vi "PH_Cam_BaseClass.ProcEvents.vi"(0 "i ref in":refnum<vi>, 5 "error in":errorcluster) -> (14 "i ref out":refnum<vi>, 19 "error out":errorcluster)   [LabVIEW 2014, in "PH_Cam_BaseClass.lvlib"]
doc: "This method is used to define the events the object will listen to. Add your own events here."
uses:
  PH_Cam_BaseClass.lvlib
  CS_Core/BaseProcess/BaseProcess.event definition.ctl
  CS_Core/CAEObj/CAEObj.event definition.ctl
  CS_Core/BaseProcess/BaseProcess.descriptor string definition.ctl
  CS_Core/BaseProcess/BaseProcess.lvlib
  CS_Core/CAEObj/CAEObj.lvlib
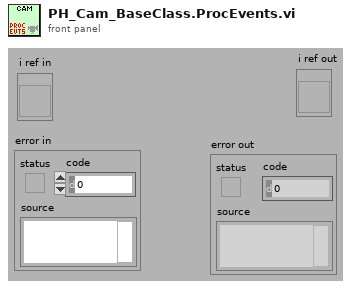
[diagram p1: front panel]
types:
  T1 = typedef "BaseProcess.lvlib/BaseProcess.event definition.ctl" = cluster{"CAEEvtDef":T2, "Data Descriptor":T3}
  T2 = typedef "CAEObj.lvlib/CAEObj.event definition.ctl" = cluster{"URL":string, "enable":bool, "ignoreResID":bool}
  T3 = typedef "BaseProcess.lvlib/BaseProcess.descriptor string definition.ctl" = string
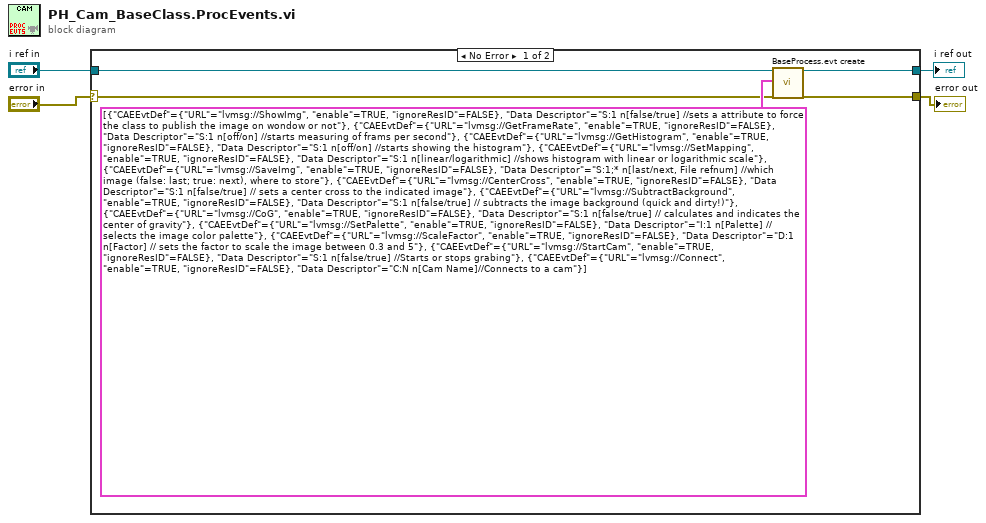
[diagram p0: block diagram]
diagram:
  n1 = case shown="No Error" "error in" {
    selector: "error in" -> [w5 w10]
    tunnel: "i ref in" -> [w6 w11]
    tunnel: [w9 w11] -> w3
    tunnel: [w8 w10] -> w2
    frame No Error {
      n2 = call "BaseProcess.evt create.vi"("i ref in"=w6, "newEvents"=T1[] [{"CAEEvtDef"={"URL"="lvmsg://ShowImg", "enable"=TRUE, "ignoreResID"=FALSE}, "Data Descriptor"="S:1 n[false/true] //sets a attribute to force the class to publish the image on wondow or not"}, {"CAEEvtDef"={"URL"="lvmsg://GetFrameRate", "enable"=TRUE, "ignoreResID"=FALSE}, "Data Descriptor"="S:1 n[off/on] //starts measuring of frams per second"}, {"CAEEvtDef"={"URL"="lvmsg://GetHistogram", "enable"=TRUE, "ignoreResID"=FALSE}, "Data Descriptor"="S:1 n[off/on] //starts showing the histogram"}, {"CAEEvtDef"={"URL"="lvmsg://SetMapping", "enable"=TRUE, "ignoreResID"=FALSE}, "Data Descriptor"="S:1 n[linear/logarithmic] //shows histogram with linear or logarithmic scale"}, {"CAEEvtDef"={"URL"="lvmsg://SaveImg", "enable"=TRUE, "ignoreResID"=FALSE}, "Data Descriptor"="S:1;* n[last/next, File refnum] //which image (false: last; true: next), where to store"}, {"CAEEvtDef"={"URL"="lvmsg://CenterCross", "enable"=TRUE, "ignoreResID"=FALSE}, "Data Descriptor"="S:1 n[false/true] // sets a center cross to the indicated image"}, {"CAEEvtDef"={"URL"="lvmsg://SubtractBackground", "enable"=TRUE, "ignoreResID"=FALSE}, "Data Descriptor"="S:1 n[false/true] // subtracts the image background (quick and dirty!)"}, {"CAEEvtDef"={"URL"="lvmsg://CoG", "enable"=TRUE, "ignoreResID"=FALSE}, "Data Descriptor"="S:1 n[false/true] // calculates and indicates the center of gravity"}, {"CAEEvtDef"={"URL"="lvmsg://SetPalette", "enable"=TRUE, "ignoreResID"=FALSE}, "Data Descriptor"="I:1 n[Palette] // selects the image color palette"}, {"CAEEvtDef"={"URL"="lvmsg://ScaleFactor", "enable"=TRUE, "ignoreResID"=FALSE}, "Data Descriptor"="D:1 n[Factor] // sets the factor to scale the image between 0.3 and 5"}, {"CAEEvtDef"={"URL"="lvmsg://StartCam", "enable"=TRUE, "ignoreResID"=FALSE}, "Data Descriptor"="S:1 n[false/true] //Starts or stops grabing"}, {"CAEEvtDef"={"URL"="lvmsg://Connect", "enable"=TRUE, "ignoreResID"=FALSE}, "Data Descriptor"="C:N n[Cam Name]//Connects to a cam"}] ("new events(V3.0)"), "error in (no error)"=w5) -> ("i ref out"=w9:refnum<vi>, "error out"=w8:errorcluster)  [unwired: 13 in, 2 out]
    }
    frame Error {
    }
  }
  "i ref out" <- w3
  "error out" <- w2
